vi "Register gRPC Methods.vi"(8 "error in (no error)":errorcluster, 11 "Template Server in":refnum<class "HVC4.lvclass">) -> (0 "error out":errorcluster, 3 "Template Server out":refnum<class "HVC4.lvclass">)   [LabVIEW 2019, in "HVC4.lvlib" / "HVC4.lvclass"]
uses:
  HVC4.lvclass
  typeDefs/Server Internal UEs.ctl
  typeDefs/Server Internal Message.ctl
  typeDefs/Server gRPC UEs.ctl
  gRPC lvSupport/Server API/typeDefs/gRPCId Cluster.ctl
  gRPC lvSupport/Server API/typeDefs/grpcId.ctl
  HVC4.lvclass/HVC4.ctl
  gRPC lvSupport/gprc-lvsupport.lvlib
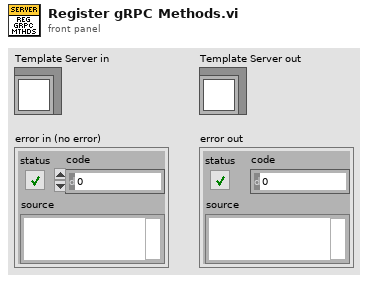
[diagram p1: front panel]
types:
  T1 = typedef "HVC4.lvlib/HVC4.lvclass/Server gRPC UEs.ctl" = cluster{"Invoke gRPC UE":refnum<user-event>, "Query gRPC UE":refnum<user-event>, "Register gRPC UE":refnum<user-event>, "ConfigureDMM gRPC UE":refnum<user-event>, "PerformDMMVoltageMeasurement gRPC UE":refnum<user-event>, "ConfigureSMU gRPC UE":refnum<user-event>, "EnableSMUOutput gRPC UE":refnum<user-event>, "DisableSMUOutput gRPC UE":refnum<user-event>, "PerformSMUCurrentMeasurement gRPC UE":refnum<user-event>}
  T2 = typedef "HVC4.lvlib/HVC4.lvclass/Server Internal UEs.ctl" = cluster{"Invoke Internal UE":refnum<user-event>, "Query Internal UE":refnum<user-event>, "Register Internal UE":refnum<user-event>, "ConfigureDMM Internal UE":refnum<user-event>, "PerformDMMVoltageMeasurement Internal UE":refnum<user-event>, "ConfigureSMU Internal UE":refnum<user-event>, "EnableSMUOutput Internal UE":refnum<user-event>, "DisableSMUOutput Internal UE":refnum<user-event>, "PerformSMUCurrentMeasurement Internal UE":refnum<user-event>}
  T3 = typedef "HVC4.lvlib/gprc-lvsupport.lvlib/grpcId.ctl" = u64
  T4 = typedef "HVC4.lvlib/HVC4.lvclass/Server Internal Message UE.ctl" = refnum<user-event>
  T5 = typedef "HVC4.lvlib/gprc-lvsupport.lvlib/gRPCId Cluster UE.ctl" = refnum<user-event>
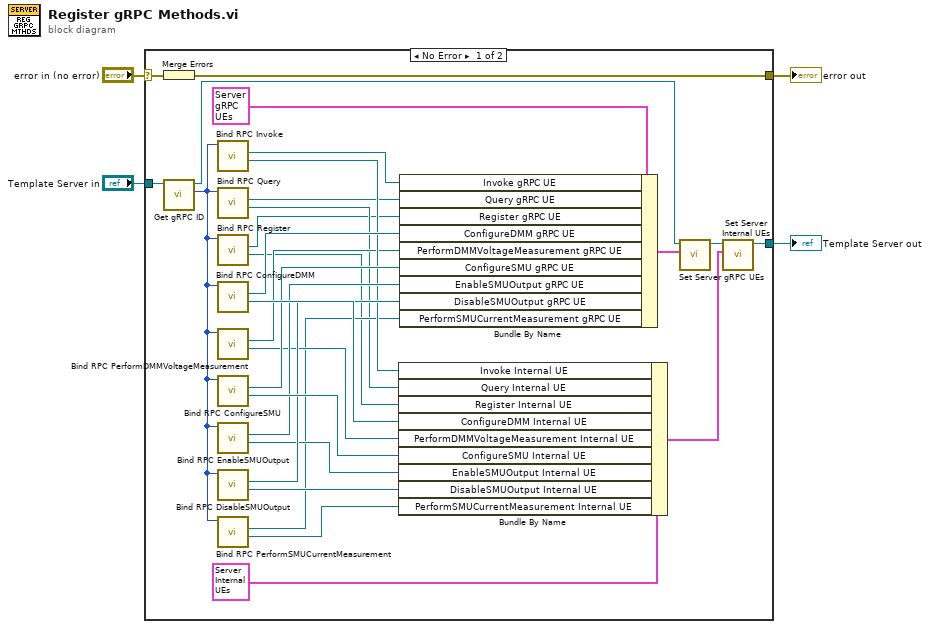
[diagram p0: block diagram]
diagram:
  n1 = case shown="No Error" "error in (no error)" {
    selector: "error in (no error)" -> [w24 w34]
    tunnel: "Template Server in" -> [w32 w35]
    tunnel: [w31 w34] -> w3
    tunnel: [w30 w35] -> w2
    frame No Error {
      n2 = Merge Errors(w24) -> (w31:errorcluster)
      n3 = call "Get gRPC ID.vi"("OOP Server in"=w32) -> ("gRPC ID"=w23:T3, "OOP Server out"=w33:refnum<class "HVC4.lvclass">)  [unwired: 9 in]
      n4 = call "Bind RPC Invoke.vi"("gRPCid server in"=w23) -> ("Invoke Internal UE"=w14:T4, "Invoke gRPC UE"=w13:T5)  [unwired: 7 in, 2 out]
      n5 = call "Bind RPC Query.vi"("gRPCid server in"=w23) -> ("Query Internal UE"=w8:T4, "Query gRPC UE"=w7:T5)  [unwired: 7 in, 2 out]
      n6 = call "Bind RPC Register.vi"("gRPCid server in"=w23) -> ("Register Internal UE"=w6:T4, "Register gRPC UE"=w5:T5)  [unwired: 7 in, 2 out]
      n7 = call "Bind RPC ConfigureDMM.vi"("gRPCid server in"=w23) -> ("ConfigureDMM Internal UE"=w22:T4, "ConfigureDMM gRPC UE"=w21:T5)  [unwired: 7 in, 2 out]
      n8 = call "Bind RPC PerformDMMVoltageMeasurement.vi"("gRPCid server in"=w23) -> ("PerformDMMVoltageMeasurement Internal UE"=w12:T4, "PerformDMMVoltageMeasurement gRPC UE"=w11:T5)  [unwired: 7 in, 2 out]
      n9 = call "Bind RPC ConfigureSMU.vi"("gRPCid server in"=w23) -> ("ConfigureSMU Internal UE"=w20:T4, "ConfigureSMU gRPC UE"=w19:T5)  [unwired: 7 in, 2 out]
      n10 = call "Bind RPC EnableSMUOutput.vi"("gRPCid server in"=w23) -> ("EnableSMUOutput Internal UE"=w16:T4, "EnableSMUOutput gRPC UE"=w15:T5)  [unwired: 7 in, 2 out]
      n11 = call "Bind RPC DisableSMUOutput.vi"("gRPCid server in"=w23) -> ("DisableSMUOutput Internal UE"=w18:T4, "DisableSMUOutput gRPC UE"=w17:T5)  [unwired: 7 in, 2 out]
      n12 = call "Bind RPC PerformSMUCurrentMeasurement.vi"("gRPCid server in"=w23) -> ("PerformSMUCurrentMeasurement Internal UE"=w10:T4, "PerformSMUCurrentMeasurement gRPC UE"=w9:T5)  [unwired: 7 in, 2 out]
      n13 = Bundle By Name ("Bundle Internal UEs")(cluster=T2 {"Invoke Internal UE"=refnum, "Query Internal UE"=refnum, "Register Internal UE"=refnum, "ConfigureDMM Internal UE"=refnum, "PerformDMMVoltageMeasurement Internal UE"=refnum, "ConfigureSMU Internal UE"=refnum, "EnableSMUOutput Internal UE"=refnum, "DisableSMUOutput Internal UE"=refnum, "PerformSMUCurrentMeasurement Internal UE"=refnum} ("Server Internal UEs"), "Invoke Internal UE"=w14, "Query Internal UE"=w8, "Register Internal UE"=w6, "ConfigureDMM Internal UE"=w22, "PerformDMMVoltageMeasurement Internal UE"=w12, "ConfigureSMU Internal UE"=w20, "EnableSMUOutput Internal UE"=w16, "DisableSMUOutput Internal UE"=w18, "PerformSMUCurrentMeasurement Internal UE"=w10) -> (w29:T2)
      n14 = Bundle By Name ("Bundle gRPC UEs")(cluster=T1 {"Invoke gRPC UE"=refnum, "Query gRPC UE"=refnum, "Register gRPC UE"=refnum, "ConfigureDMM gRPC UE"=refnum, "PerformDMMVoltageMeasurement gRPC UE"=refnum, "ConfigureSMU gRPC UE"=refnum, "EnableSMUOutput gRPC UE"=refnum, "DisableSMUOutput gRPC UE"=refnum, "PerformSMUCurrentMeasurement gRPC UE"=refnum} ("gRPC Server Method Events"), "Invoke gRPC UE"=w13, "Query gRPC UE"=w7, "Register gRPC UE"=w5, "ConfigureDMM gRPC UE"=w21, "PerformDMMVoltageMeasurement gRPC UE"=w11, "ConfigureSMU gRPC UE"=w19, "EnableSMUOutput gRPC UE"=w15, "DisableSMUOutput gRPC UE"=w17, "PerformSMUCurrentMeasurement gRPC UE"=w9) -> (w26:T1)
      n15 = call "Set Server gRPC UEs.vi"("Server gRPC UEs"=w26, "OOP Server in"=w33) -> ("OOP Server out"=w27:refnum<class "HVC4.lvclass">)  [unwired: 9 in]
      n16 = call "Set Server Internal UEs.vi"("Server Internal UEs"=w29, "OOP Server in"=w27) -> ("OOP Server out"=w30:refnum<class "HVC4.lvclass">)  [unwired: 9 in]
    }
    frame Error {
    }
  }
  "error out" <- w3
  "Template Server out" <- w2
